vi "Test_Main.vi"() -> ()   [LabVIEW 2025]
doc: "Demonstrates how to use the DC Voltage Output Function to force an output voltage. This example initializes a session, configures the Output Function, Sense, Autorange, Voltage Level and Current Limit, initiates generation, waits for a specified delay, and measures the voltage and current output. This example uses Single Point source mode."
uses:
  <instrlib>/niDCPower/nidcpower.llb/niDCPower Source Mode.ctl
  <instrlib>/niDCPower/nidcpower.llb/niDCPower Wait For Event - Event.ctl
  <instrlib>/niDCPower/nidcpower.llb/niDCPower Output Function.ctl
  <instrlib>/niDCPower/nidcpower.llb/niDCPower Get Channel Name From String.vi
panel:
  in  "Source Delay (Sec)":dbl=0.1 format="%.3p"
  out "Voltage Measurement":dbl
  out "Current Measurement":dbl
  in  "Current Limit Range":dbl=0.1 format="%.3p"
  in  "Voltage Level Range":dbl=6.0 format="%.5p"
  out "Compliance/Limit Reached":bool
  in  "Current Limit":dbl=0.06 format="%.3p"
  in  "Voltage Level":dbl=2.0 format="%.5p"
  in  "Resource Name":refnum<k15>="Dev1"
  # "Overview: Demonstrates how to use the DC Voltage Output Function to force an output voltage.  \nThis example initializes a session; configures the Output Function, Voltage Level and Current Limit; \ninitiates generation; waits for a specified delay; and measures the voltage and current output. \nRequirements: NI-DCPower\nInstructions:\n1. Specify the appropriate instrument channel in the Resource Name control.\n2. Configure the parameters of the DC Voltage signal you'd like to output.\n3. Run the VI."
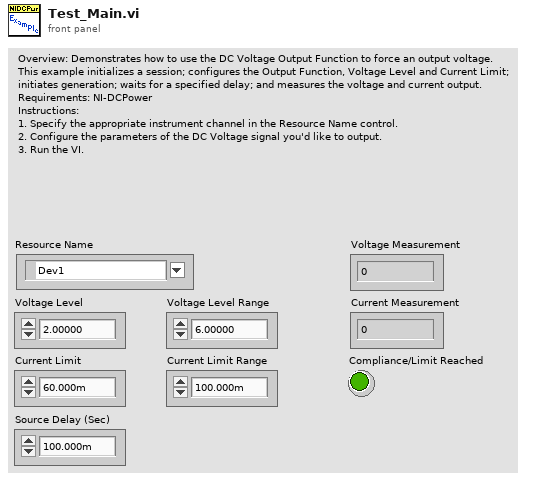
[diagram p1: front panel]
types:
  T1 = typedef "niDCPower Output Function.ctl" = i32
  T2 = typedef "niDCPower Wait For Event - Event.ctl" = i32
  T3 = typedef "niDCPower Source Mode.ctl" = i32
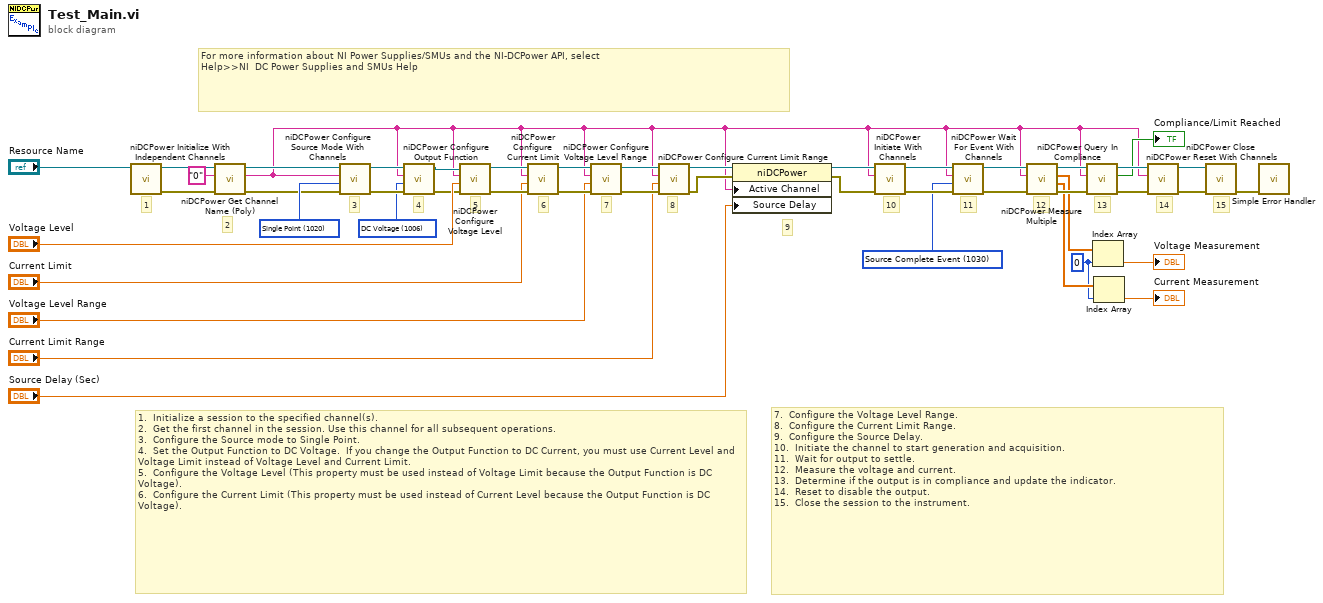
[diagram p0: block diagram]
diagram:
  w6 = T1 1006 items=["DC Voltage"=1006, "DC Current"=1007, "Pulse Voltage"=1049, "Pulse Current"=1050] ("output function")
  w10 = T2 1030 items=["Source Complete Event"=1030, "Measure Complete Event"=1031, "Sequence Iteration Complete Event"=1032, "Sequence Engine Done Event"=1033] ("event")
  w22 = 0 ("index")
  w33 = T3 1020 items=["Single Point"=1020, "Sequence"=1021] ("source mode")
  # "2"
  # "For more information about NI Power Supplies/SMUs and the NI-DCPower API, select\nHelp>>NI  DC Power Supplies and SMUs Help"
  # "15"
  # "10"
  # "12"
  # "11"
  # "8"
  # "7"
  # "3"
  # "1.  Initialize a session to the specified channel(s).\n2.  Get the first channel in the session. Use this channel for all subsequent operations.\n3.  Configure the Source mode to Single Point.\n4.  Set the Output Function to DC Voltage.  If you change the Output Function to DC Current, you must use Current Level and Voltage Limit instead of Voltage Level and Current Limit.\n5.  Configure the Voltage Level (This property must be used instead of Voltage Limit because the Output Function is DC Voltage).\n6.  Configure the Current Limit (This property must be used instead of Current Level because the Output Function is DC Voltage)."
  # "4"
  # "13"
  # "7.  Configure the Voltage Level Range.\n8.  Configure the Current Limit Range.\n9.  Configure the Source Delay.\n10.  Initiate the channel to start generation and acquisition.\n11.  Wait for output to settle.\n12.  Measure the voltage and current.\n13.  Determine if the output is in compliance and update the indicator.\n14.  Reset to disable the output.\n15.  Close the session to the instrument."
  # "14"
  # "9"
  # "6"
  # "5"
  # "1"
  n1 = call <instrlib>:"niDCPower Initialize With Independent Channels.vi"("resource name"="Resource Name") -> ("error out"=w3:errorcluster, "instrument handle out"=w36:refnum<k15>)  [unwired: 9 in]
  n2 = call-poly <instrlib>:"niDCPower Get Channel Name (Poly).vi"("error in (no error)"=w3, "index"="0", "instrument handle"=w36) -> ("error out"=w2:errorcluster, "name"=w1:string, "instrument handle out"=w5:refnum<k15>)  [unwired: 6 in]
  n3 = call <instrlib>:"niDCPower Configure Source Mode With Channels.vi"("error in (no error)"=w2, "source mode"=w33, "channel name"=w1, "instrument handle"=w5) -> ("error out"=w35:errorcluster, "instrument handle out"=w34:refnum<k15>)  [unwired: 6 in]
  n4 = call <instrlib>:"niDCPower Configure Output Function.vi"("error in (no error)"=w35, "output function"=w6, "channel name"=w1, "instrument handle"=w34) -> ("error out"=w8:errorcluster, "instrument handle out"=w9:refnum<k15>)  [unwired: 6 out]
  n5 = call <instrlib>:"niDCPower Configure Voltage Level.vi"("error in (no error)"=w8, "voltage level"="Voltage Level", "channel name"=w1, "instrument handle"=w9) -> ("error out"=w44:errorcluster, "instrument handle out"=w45:refnum<k15>)  [unwired: 6 out]
  n6 = call <instrlib>:"niDCPower Configure Current Limit.vi"("error in (no error)"=w44, "current limit"="Current Limit", "channel name"=w1, "instrument handle"=w45) -> ("error out"=w32:errorcluster, "instrument handle out"=w31:refnum<k15>)  [unwired: 1 in, 5 out]
  n7 = call <instrlib>:"niDCPower Configure Voltage Level Range.vi"("error in (no error)"=w32, "voltage level range"="Voltage Level Range", "channel name"=w1, "instrument handle"=w31) -> ("error out"=w30:errorcluster, "instrument handle out"=w29:refnum<k15>)  [unwired: 6 out]
  n8 = call <instrlib>:"niDCPower Configure Current Limit Range.vi"("error in (no error)"=w30, "current limit range"="Current Limit Range", "channel name"=w1, "instrument handle"=w29) -> ("error out"=w16:errorcluster, "instrument handle out"=w19:refnum<k15>)  [unwired: 6 out]
  n9 = property class="niDCPower"(reference=w19, error in=w16, "Active Channel"=w1, "Source Delay"="Source Delay (Sec)") -> (reference out=w18:refnum<k15>, error out=w17:errorcluster)
  n10 = call <instrlib>:"niDCPower Initiate With Channels.vi"("error in (no error)"=w17, "channel name"=w1, "instrument handle"=w18) -> ("error out"=w12:errorcluster, "instrument handle out"=w14:refnum<k15>)  [unwired: 7 in]
  n11 = call <instrlib>:"niDCPower Wait For Event With Channels.vi"("error in (no error)"=w12, "event"=w10, "channel name"=w1, "instrument handle"=w14) -> ("error out"=w11:errorcluster, "instrument handle out"=w13:refnum<k15>)  [unwired: 6 in]
  n12 = call <instrlib>:"niDCPower Measure Multiple.vi"("error in (no error)"=w11, "channel name"=w1, "instrument handle"=w13) -> ("error out"=w25:errorcluster, "current measurements"=w23:dbl[], "voltage measurements"=w24:dbl[], "instrument handle out"=w26:refnum<k15>)  [unwired: 5 out]
  n13 = call <instrlib>:"niDCPower Query In Compliance.vi"("error in (no error)"=w25, "channel name"=w1, "instrument handle"=w26) -> ("error out"=w39:errorcluster, "in compliance?"=→"Compliance/Limit Reached":bool, "instrument handle out"=w42:refnum<k15>)  [unwired: 6 out]
  n14 = Index Array(array=w24, index=w22) -> (element=→"Voltage Measurement":dbl)
  n15 = Index Array(array=w23, index=w22) -> (element=→"Current Measurement":dbl)
  n16 = call <instrlib>:"niDCPower Reset With Channels.vi"("error in (no error)"=w39, "channel name"=w1, "instrument handle"=w42) -> ("error out"=w40:errorcluster, "instrument handle out"=w41:refnum<k15>)  [unwired: 7 in]
  n17 = call <instrlib>:"niDCPower Close.vi"("error in (no error)"=w40, "instrument handle"=w41) -> ("error out"=w38:errorcluster)  [unwired: 9 out]
  n18 = call <vilib>:"Simple Error Handler.vi"("error in (no error)"=w38) -> ()  [unwired: 1 in, 8 out]
